vi "Get BC.vi"(8 "error in (no error)":errorcluster, 10 "Domain":refnum<class "NI_Domain.lvclass">, 11 "BC_Evolut_1D_Numeric in":refnum<class "NI_BC_Evolut_1D_Numeric.lvclass">) -> (0 "error out":errorcluster, 2 "BC":variant, 3 "BC_Evolut_1D_Numeric out":refnum<class "NI_BC_Evolut_1D_Numeric.lvclass">)   [LabVIEW 2017, in "NI_PDE.lvlib" / "NI_BC_Evolut_1D_Numeric.lvclass"]
uses:
  <vilib>/gmath/pde.llb/BCClass/BC_Evolut_1D_Numeric/NI_BC_Evolut_1D_Numeric.lvclass
  <vilib>/gmath/pde.llb/DomainClass/NI_Domain.lvclass
  <vilib>/gmath/pde.llb/Common/PDE_BC Type.ctl
  <vilib>/gmath/pde.llb/Common/PDE_BC Position 1D.ctl
  <vilib>/gmath/pde.llb/BCClass/BC_Evolut_1D_Numeric/NI_BC_Evolut_1D_Numeric.lvclass/NI_BC_Evolut_1D_Numeric.ctl
  <vilib>/gmath/NI_PDE.lvlib
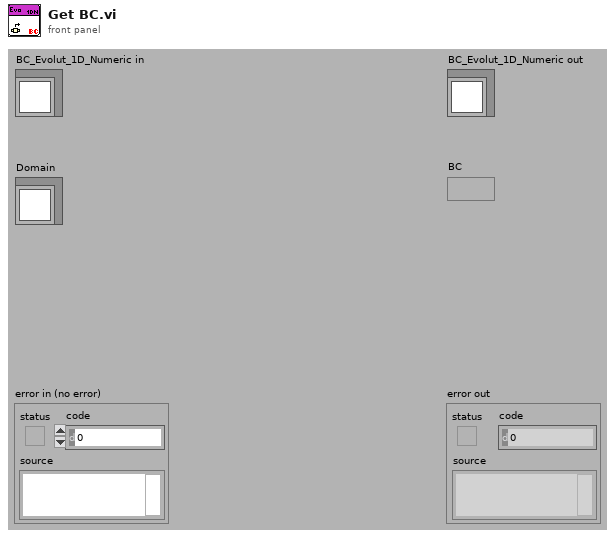
[diagram p1: front panel]
types:
  T1 = typedef "NI_PDE.lvlib/PDE_BC Type.ctl" = i32
  T2 = typedef "NI_PDE.lvlib/PDE_BC Position 1D.ctl" = i32
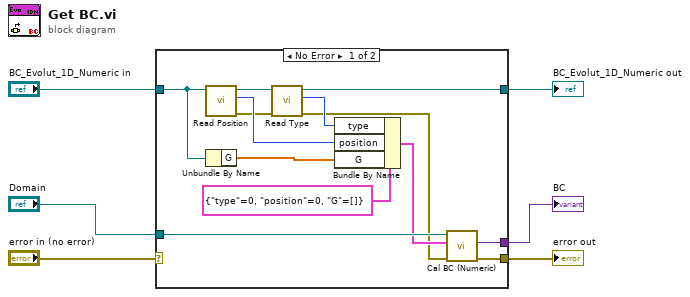
[diagram p0: block diagram]
diagram:
  n1 = case shown="No Error" "error in (no error)" {
    selector: "error in (no error)" -> [_ w20]
    tunnel: "BC_Evolut_1D_Numeric in" -> [w18 w21]
    tunnel: [w9 _] -> w4
    tunnel: [w8 w20] -> w5
    tunnel: [w17 w21] -> w3
    tunnel: "Domain" -> [w11 _]
    frame No Error {
      n2 = call-dynamic "Read Position.vi"("BC_Evolut_1D.lvclass in"=w18) -> ("error out"=w12:errorcluster, "BC position 1D"=w14:T2, "BC_Evolut_1D.lvclass out"=w19:refnum<class "NI_BC_Evolut_1D_Numeric.lvclass">)  [unwired: 1 in, 7 out]
      n3 = Unbundle By Name(w18) -> ("G"=w13:dbl[])
      n4 = call-dynamic "Read Type.vi"("error in (no error)"=w12, "BC.lvclass in"=w19) -> ("error out"=w7:errorcluster, "BC type"=w15:T1, "BC.lvclass out"=w17:refnum<class "NI_BC_Evolut_1D_Numeric.lvclass">)  [unwired: 7 out]
      n5 = Bundle By Name(cluster=cluster{"type":T1, "position":T2, "G":dbl[]} {"type"=0, "position"=0, "G"=[]} ("BC data"), "type"=w15, "position"=w14, "G"=w13) -> (w10:cluster{"type":T1, "position":T2, "G":dbl[]})
      n6 = call-dynamic "Cal BC (Numeric).vi"("error in (no error)"=w7, "BC in"=w10, "Domain in"=w11) -> ("error out"=w8:errorcluster, "BC out"=w9:variant)  [unwired: 7 out]
    }
    frame Error {
    }
  }
  "BC" <- w4
  "error out" <- w5
  "BC_Evolut_1D_Numeric out" <- w3
